vi "swap.vi"(8 "error in (no error)":errorcluster, 10 "storage type target":T1, 11 "Image in":refnum<class "Image.lvclass">) -> (0 "error out":errorcluster, 3 "Image out":refnum<class "Image.lvclass">, 4 "previous storage mode":T1)   [LabVIEW 2010, in "Image.lvclass"]
uses:
  Image.lvclass
  storage_mode.ctl
  target_format_enum.ctl
  ErrorController/ErrorController/class_data.vi
  ErrorController/ErrorController/ErrorController.lvclass
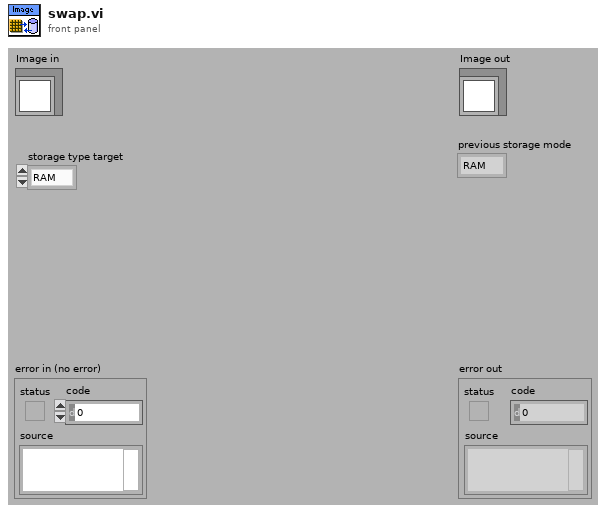
[diagram p1: front panel]
types:
  T1 = typedef "Image.lvclass/storage_mode.ctl" = enum16{"RAM", "disk"}
  T2 = typedef "target_format_enum.ctl" = enum16{"don't force", "uint8", "uint16", "int16", "uint32", "int32", "single float"}
  T3 = typedef "Image Type" = u32
  T4 = typedef "IMAQ Image.ctl" = refnum<image>
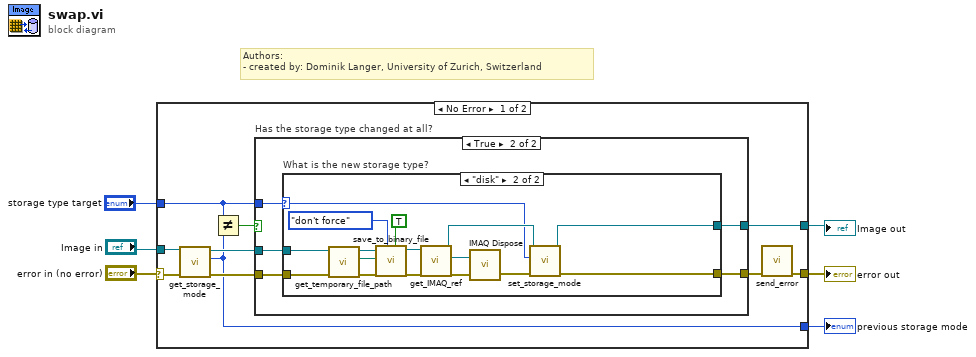
[diagram p0: block diagram]
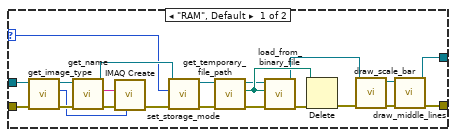
[diagram p3: hidden frame]
diagram:
  # "Authors: \n- created by: Dominik Langer, University of Zurich, Switzerland"
  n1 = case shown="No Error" "error in (no error)" {
    selector: "error in (no error)" -> [w13 w63]
    tunnel: [w8 w63] -> w2
    tunnel: [w11 w62] -> w3
    tunnel: "Image in" -> [w12 w62]
    tunnel: "storage type target" -> [w10 _]
    tunnel: [w9 _] -> w1
    frame No Error {
      n2 = call-dynamic "get_storage_mode.vi"("error in (no error)"=w13, "Image.lvclass in"=w12) -> ("error out"=w15:errorcluster, "storage mode"=w9:T1, "Image.lvclass out"=w14:refnum<class "Image.lvclass">)  [unwired: 7 out]
      n3 = Not Equal?(x=w10, y=w9) -> (x != y?=w16:bool)
      n4 = case "Has the storage type changed at all?" shown="True" w16 {
        tunnel: w10 -> [_ w21]
        tunnel: [w18 w20] -> w11
        tunnel: [w17 w19] -> w7
        tunnel: w14 -> [w18 w23]
        tunnel: w15 -> [w17 w22]
        frame False {
          # "The SwapImage already is in the right storage mode --> there is nothing we need to do..."
        }
        frame True {
          n5 = case "What is the new storage type?" shown="\"disk\"" w21 {
            selector: w21 -> [w30 w48]
            tunnel: w22 -> [w38 w57]
            tunnel: w23 -> [w41 w56]
            tunnel: [w24 w51] -> w20
            tunnel: [w26 w49] -> w19
            frame "RAM", Default {
              n6 = call-dynamic "get_image_type.vi"("error in (no error)"=w38, "Image.lvclass in"=w41) -> ("error out"=w39:errorcluster, "Image Type"=w35:T3, "Image.lvclass out"=w40:refnum<class "Image.lvclass">)  [unwired: 7 out]
              n7 = call-dynamic "get_name.vi"("error in (no error)"=w39, "Image in"=w40) -> ("error out"=w37:errorcluster, "name"=w36:string, "Image out"=w32:refnum<class "Image.lvclass">)  [unwired: 7 out]
              n8 = call "IMAQ Create"("Image Name"=w36, "Image Type"=w35, "error in (no error)"=w37) -> ("error out"=w34:errorcluster)  [unwired: 1 in, 2 out]
              n9 = call-dynamic "set_storage_mode.vi"("error in (no error)"=w34, "storage type"=w30, "Image.lvclass in"=w32) -> ("error out"=w33:errorcluster, "Image.lvclass out"=w31:refnum<class "Image.lvclass">)  [unwired: 7 out]
              n10 = call-dynamic "get_temporary_file_path.vi"("error in (no error)"=w33, "Image.lvclass in"=w31) -> ("error out"=w44:errorcluster, "temporary file path"=w43:path, "Image.lvclass out"=w42:refnum<class "Image.lvclass">)  [unwired: 7 out]
              n11 = call-dynamic "load_from_binary_file.vi"("error in (no error)"=w44, "Path"=w43, "Image in"=w42) -> ("error out"=w45:errorcluster, "Image out"=w28:refnum<class "Image.lvclass">)  [unwired: 7 out]
              n12 = Delete(path (use dialog)=w43, error in=w45) -> (error out=w29:errorcluster)  [unwired: 5 out]
              n13 = call "draw_scale_bar.vi"("error in (no error)"=w29, "Image in"=w28) -> ("error out"=w27:errorcluster, "Image out"=w25:refnum<class "Image.lvclass">)  [unwired: 3 in, 5 out]
              n14 = call "draw_middle_lines.vi"("error in (no error)"=w27, "Image in"=w25) -> ("error out"=w26:errorcluster, "Image out"=w24:refnum<class "Image.lvclass">)  [unwired: 1 in, 7 out]
            }
            frame "disk" {
              n15 = call-dynamic "get_temporary_file_path.vi"("error in (no error)"=w57, "Image.lvclass in"=w56) -> ("error out"=w54:errorcluster, "temporary file path"=w53:path, "Image.lvclass out"=w55:refnum<class "Image.lvclass">)  [unwired: 7 out]
              n16 = call-dynamic "save_to_binary_file.vi"("prepend array size?"=TRUE, "force format?"=target_format_enum."don't force", "error in (no error)"=w54, "Path"=w53, "Image in"=w55) -> ("error out"=w61:errorcluster, "Image out"=w60:refnum<class "Image.lvclass">)  [unwired: 3 in, 2 out]
              n17 = call-dynamic "get_IMAQ_ref.vi"("error in (no error)"=w61, "Image.lvclass in"=w60) -> ("error out"=w58:errorcluster, "Image"=w59:T4, "Image.lvclass out"=w52:refnum<class "Image.lvclass">)  [unwired: 7 out]
              n18 = call "IMAQ Dispose"("Image"=w59, "error in (no error)"=w58) -> ("error out"=w50:errorcluster)  [unwired: 1 in, 3 out]
              n19 = call-dynamic "set_storage_mode.vi"("error in (no error)"=w50, "storage type"=w48, "Image.lvclass in"=w52) -> ("error out"=w49:errorcluster, "Image.lvclass out"=w51:refnum<class "Image.lvclass">)  [unwired: 7 out]
            }
          }
        }
      }
      n20 = call "send_error.vi"("error in (no error)"=w7) -> ("error out"=w8:errorcluster)  [unwired: 10 in]
    }
    frame Error {
    }
  }
  "error out" <- w2
  "Image out" <- w3
  "previous storage mode" <- w1
